vi "Autonomous.vi"   [LabVIEW 2019]
doc: "This VI starts when autonomous period begins, and will automatically be terminated when it ends. You can carry out timed or sensor driven operations directly to I/O or to subsystems without needing to return to the caller."
uses:
  AutonBuilder/Typedef/Single Sequence.ctl
  AutonBuilder/Typedef/Sequence Command.ctl
  AutonBuilder/Typedef/Plate Arrangement.ctl
  <vilib>/Rock Robotics/Network Tables/NT Read String.vi
  Auton/Auton Kill Switch.vi
  <vilib>/Rock Robotics/Network Tables/NT Read Raw.vi
  Auton/Command Parser/Active Command.vi
types:
  T1 = typedef "Single Sequence.ctl" = cluster{"Sequence Array":T2[]}
  T2 = typedef "Sequence Command.ctl" = cluster{"Sequence Name":string, "Plate Arrangement":T3, "Command Name":string, "Data":variant, "Sequence Number":u32}
  T3 = typedef "Plate Arrangement.ctl" = cluster{"LR*":bool, "LL*":bool, "RL*":bool, "RR*":bool}
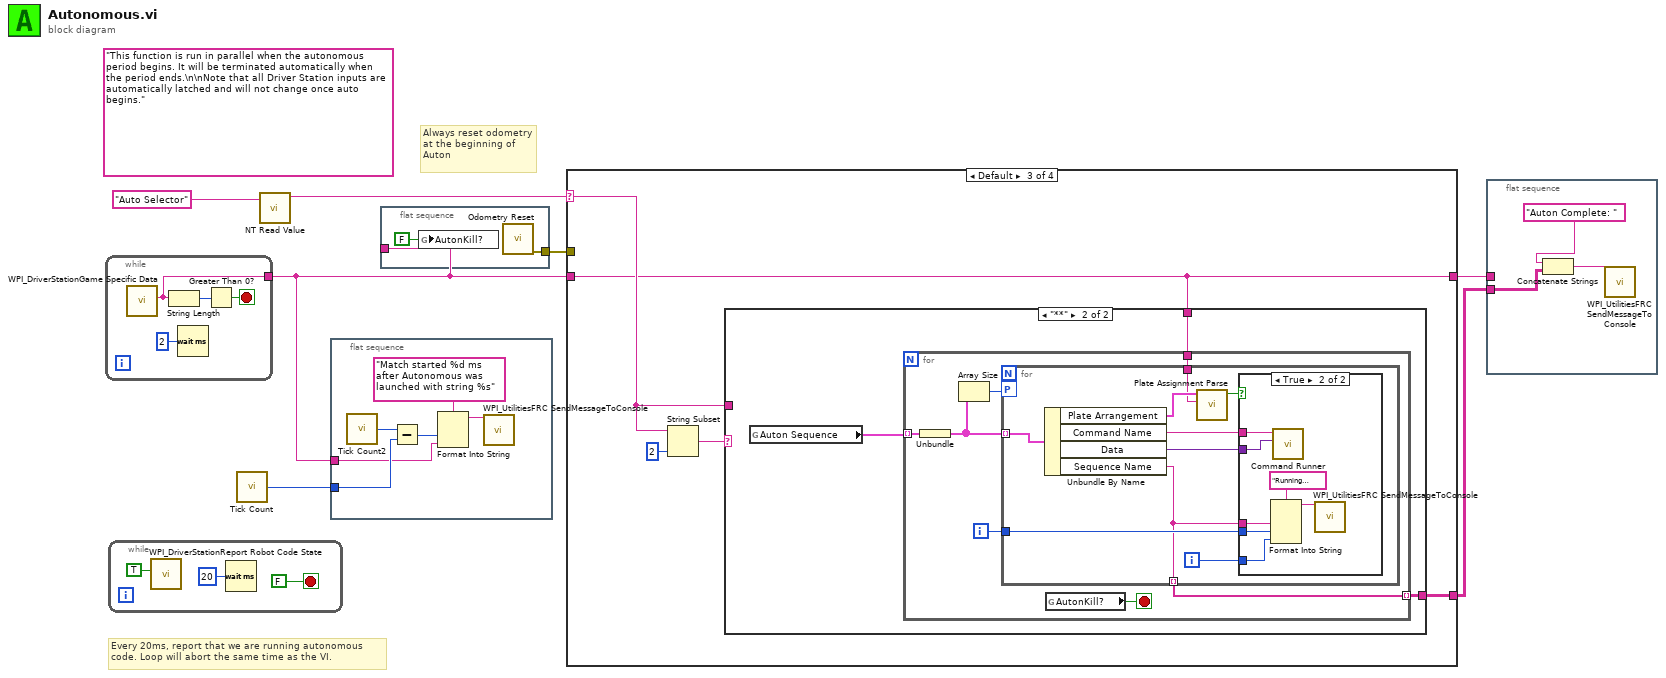
[diagram p0: block diagram]
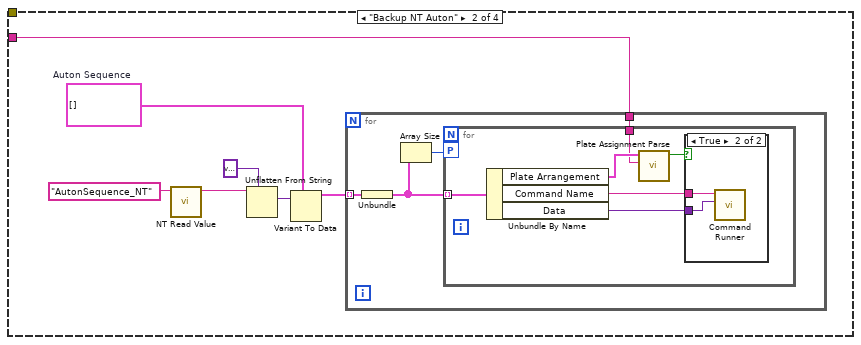
[diagram p3: hidden frame]
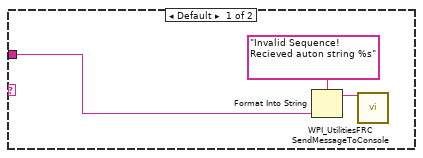
[diagram p5: hidden frame]
diagram:
  (unwired) "This function is run in parallel when the autonomous period begins. It will be terminated automatically when the period ends.\n\nNote that all Driver Station inputs are automatically latched and will not change once auto begins."
  # "Always reset odometry at the beginning of Auton"
  # "Every 20ms, report that we are running autonomous\ncode. Loop will abort the same time as the VI."
  n1 = while {
    tunnel: [w8] -> w4
    stop <- w9 stop-if-true
    n2 = call <vilib>:"WPI_DriverStationGame Specific Data.vi"() -> ("Game Specific Data"=w8:string)  [unwired: 11 in]
    n3 = String Length(string=w8) -> (length=w10:i32)
    n4 = Wait (ms)(milliseconds to wait=u32 2) -> ()  [unwired: 1 out]
    n5 = Greater Than 0?(x=w10) -> (x > 0?=w9:bool)
  }
  n6 = while {
    stop <- FALSE stop-if-true
    n7 = call <vilib>:"WPI_DriverStationReport Robot Code State.vi"("Autonomous"=TRUE) -> ()  [unwired: 10 in, 1 out]
    n8 = Wait (ms)(milliseconds to wait=u32 20) -> ()  [unwired: 1 out]
  }
  n9 = call "Tick Count"() -> ("Tick Count(mSec)"=w5:u32)
  n10 = call-poly <vilib>:"NT Read Value.vi"("Name"="Auto Selector") -> ("String"=w6:string)  [unwired: 9 in, 1 out]
  n11 = flat-sequence {
    tunnel: w5 -> [w19]
    tunnel: w4 -> [w15]
    frame #0 {
      n12 = call "Tick Count2"() -> ("Tick Count(mSec)"=w20:u32)
      n13 = Subtract(x=w20, y=w19) -> (x-y=w18:u32)
      n14 = Format Into String(format string="Match started %d ms after Autonomous was launched with string %s", w18, w15) -> (resulting string=w16:string)  [unwired: 2 in, 1 out]
      n15 = call <vilib>:"WPI_UtilitiesFRC SendMessageToConsole.vi"("Message"=w16) -> ()  [unwired: 14 in, 1 out]
    }
  }
  n16 = flat-sequence {
    tunnel: w4 -> [_]
    tunnel: [w22] -> w3
    frame #0 {
      n17 = global write "Auton Kill Switch.vi" "AutonKill?"(FALSE ("AutonKill?")) -> ()
      n18 = call "Odometry Reset.vi"() -> ("error out"=w22:errorcluster)  [unwired: 11 in]
    }
  }
  n19 = case shown="Default" w6 {
    selector: w6 -> [_ _ w46 _]
    tunnel: w4 -> [_ w23 w43 _]
    tunnel: w3 -> [_ _ _ _]
    tunnel: [_ _ w43 _] -> w2
    tunnel: [_ _ w42 _] -> w1
    frame "Alternative 1" {
    }
    frame "Backup NT Auton" {
      w25 = T1[] []  # Auton Sequence
      n20 = call-poly <vilib>:"NT Read Value.vi"("Name"="AutonSequence_NT") -> ("Raw"=w28:string)  [unwired: 9 in, 1 out]
      n21 = Unflatten From String(type=variant, binary string=w28) -> (value=w26:variant)  [unwired: 3 in, 2 out]
      n22 = Variant To Data(type=w25, Variant=w26) -> (data=w24:T1[])  [unwired: 1 in, 1 out]
      n23 = for {
        tunnel: w24 -> [w32] mode=indexing
        tunnel: w23 -> [w30]
        n24 = Unbundle(w32) -> ("Sequence Array"=w31:T2[])
        n25 = Array Size(array=w31) -> (size(s)=w33:i32)
        n26 = for {
          workers-P: w33 -> [_]
          tunnel: w31 -> [w39] mode=indexing
          tunnel: w30 -> [w37]
          n27 = Unbundle By Name(w39) -> ("Plate Arrangement"=w38:T3, "Command Name"=w35:string, "Data"=w34:variant)
          n28 = call "Plate Assignment Parse.vi"("Game String"=w37, "Plate Arrangement"=w38) -> ("Match?"=w36:bool)  [unwired: 9 in]
          n29 = case shown="True" w36 {
            tunnel: w35 -> [_ w41]
            tunnel: w34 -> [_ w40]
            frame False {
            }
            frame True {
              n30 = call "Command Runner.vi"("Data"=w40, "Command Name"=w41) -> ()  [unwired: 10 in]
            }
          }
        }
      }
    }
    frame Default {
      n31 = String Subset(string=w46, length (rest)=2 ("length (rest)")) -> (substring=w44:string)  [unwired: 1 in]
      n32 = case shown="\"**\"" w44 {
        tunnel: w43 -> [_ w52]
        tunnel: w46 -> [w47 _]
        tunnel: [_ w50] -> w42
        frame Default {
          n33 = Format Into String(format string="Invalid Sequence! Recieved auton string %s", w47) -> (resulting string=w49:string)  [unwired: 2 in, 1 out]
          n34 = call <vilib>:"WPI_UtilitiesFRC SendMessageToConsole.vi"("Message"=w49) -> ()  [unwired: 14 in, 1 out]
        }
        frame "**" {
          n35 = global read "Active Command.vi" "Auton Sequence"() -> (w51:T1[])
          n36 = for {
            tunnel: w51 -> [w59] mode=indexing
            tunnel: w52 -> [w57]
            tunnel: [w54] -> w50 mode=indexing
            i -> [w56]
            stop <- w53 stop-if-true
            n37 = Unbundle(w59) -> ("Sequence Array"=w58:T2[])
            n38 = Array Size(array=w58) -> (size(s)=w55:i32)
            n39 = for {
              tunnel: w58 -> [w68] mode=indexing
              tunnel: w57 -> [w66]
              tunnel: w56 -> [w62]
              workers-P: w55 -> [_]
              tunnel: [w60] -> w54 mode=indexing
              i -> [w61]
              n40 = Unbundle By Name(w68) -> ("Plate Arrangement"=w67:T3, "Command Name"=w64:string, "Data"=w63:variant, "Sequence Name"=w60:string)
              n41 = call "Plate Assignment Parse.vi"("Game String"=w66, "Plate Arrangement"=w67) -> ("Match?"=w65:bool)  [unwired: 9 in]
              n42 = case shown="True" w65 {
                tunnel: w64 -> [_ w75]
                tunnel: w63 -> [_ w74]
                tunnel: w60 -> [_ w71]
                tunnel: w62 -> [_ w70]
                tunnel: w61 -> [_ w69]
                frame False {
                }
                frame True {
                  n43 = Format Into String(format string="Running command %s, sequence %d, number in sequence %d", w71, w70, w69) -> (resulting string=w73:string)  [unwired: 2 in, 1 out]
                  n44 = call "Command Runner.vi"("Data"=w74, "Command Name"=w75) -> ()  [unwired: 10 in]
                  n45 = call <vilib>:"WPI_UtilitiesFRC SendMessageToConsole.vi"("Message"=w73) -> ()  [unwired: 14 in, 1 out]
                }
              }
            }
            n46 = global read "Auton Kill Switch.vi" "AutonKill?"() -> (w53:bool)
          }
        }
      }
    }
    frame "Alternative 2" {
    }
  }
  n47 = flat-sequence {
    tunnel: w2 -> [_]
    tunnel: w1 -> [w77]
    frame #0 {
      n48 = Concatenate Strings("Auton Complete: " ("Message"), w77) -> (w76:string)
      n49 = call <vilib>:"WPI_UtilitiesFRC SendMessageToConsole.vi"("Message"=w76) -> ()  [unwired: 14 in, 1 out]
    }
  }
